vi "Launch Valves.vi"(8 "error in (no error)":errorcluster, 11 "Sample Line in":refnum<class "Sample Line.lvclass">) -> (0 "error out":errorcluster, 3 "Sample Line out":refnum<class "Sample Line.lvclass">)   [LabVIEW 2015, in "cRIO-Carbondioxide.lvlib" / "CO2-Actor.lvlib" / "Sample Line.lvclass"]
doc: "(<B>Filename</B>: Actor Framework.lvlib:Actor.lvclass:Pre Launch Init.vi)\n\nDefines behavior that occurs after the Launch Actor method is invoked but before the actor's Actor Core method begins running.\n\nThe Pre Launch Init method is guaranteed to finish before the Launch Actor method returns to its caller and before the actor itself receives any messages. Any references that the Pre Launch Init method obtains are guaranteed to have the same lifetime as the actor itself. Any errors that the Pre Launch Init method returns will abort the launch.\n\nBy default, this method does nothing. A descendant class may override it to define behavior."
uses:
  Sample Line.lvclass
  Valve/Action.ctl
  <vilib>/ActorFramework/Actor/Actor.lvclass
  Sample Line.lvclass/Sample Line.ctl
  CO2 Actor/CO2 Actor.lvclass
  Valve/Valve.lvclass
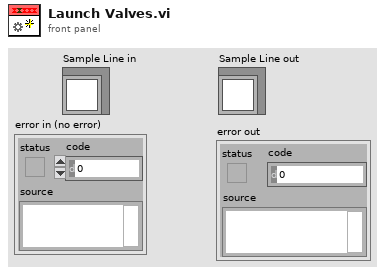
[diagram p1: front panel]
types:
  T1 = typedef "Action.ctl" = enum16{"Open", "Close", "None"}
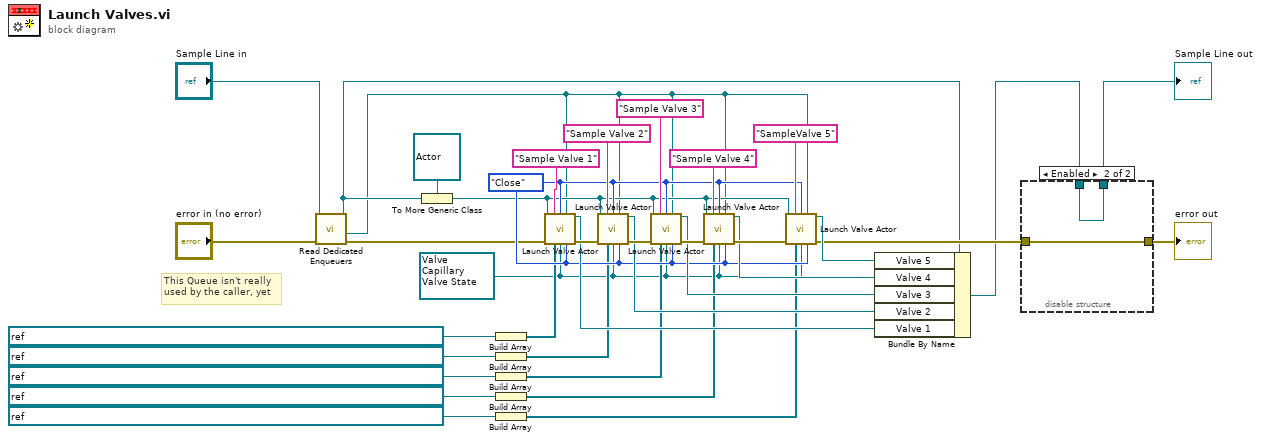
[diagram p0: block diagram]
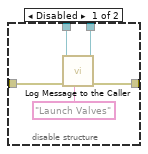
[diagram p2: hidden frame]
diagram:
  w3 = refnum<queue> refnum ("StateQ")
  w18 = Action."Close" ("Start Action (Open)")
  # "This Queue isn't really\nused by the caller, yet"
  n1 = call "Read Dedicated Enqueuers.vi"("error in (no error)"="error in (no error)", "CO2 Actor in"="Sample Line in") -> ("error out"=w5:errorcluster, "DedicatedEnQrs"=w1:refnum<queue>, "CO2 Actor out"=w2:refnum<class "Sample Line.lvclass">)  [unwired: 6 in, 1 out]
  n2 = To More Generic Class(target class=refnum<class "Actor.lvclass"> refnum ("Caller Actor in"), reference=w2) -> (generic class reference=w8:refnum<class "Actor.lvclass">)
  n3 = Build Array(refnum<k21> "ni.var.psp://10.2.0.20/AMS Gas SHV/Valves/Sample Line Valves/Sample Line 1" ("SHV")) -> (w13:refnum<k21>[])
  n4 = Build Array(refnum<k21> "ni.var.psp://10.2.0.20/AMS Gas SHV/Valves/Sample Line Valves/Sample Line 2" ("SHV")) -> (w12:refnum<k21>[])
  n5 = Build Array(refnum<k21> "ni.var.psp://10.2.0.20/AMS Gas SHV/Valves/Sample Line Valves/Sample Line 3" ("SHV")) -> (w11:refnum<k21>[])
  n6 = Build Array(refnum<k21> "ni.var.psp://10.2.0.20/AMS Gas SHV/Valves/Sample Line Valves/Sample Line 4" ("SHV")) -> (w10:refnum<k21>[])
  n7 = Build Array(refnum<k21> "ni.var.psp://10.2.0.20/AMS Gas SHV/Valves/Sample Line Valves/Sample Line 5" ("SHV")) -> (w9:refnum<k21>[])
  n8 = call "Launch Valve Actor.vi"("Caller Actor in"=w8, "Name"="Sample Valve 1", "Start Action (Open)"=w18, "DedicatedEnQrs"=w1, "error in (no error)"=w5, "SHV"=w13, "StateQ"=w3, "Stop Action (Close)"=w18) -> ("Caller-To-Actor Enqueuer"=w23:refnum<class "Message Enqueuer.lvclass">, "error out"=w36:errorcluster)  [unwired: 6 in]
  n9 = call "Launch Valve Actor.vi"("Caller Actor in"=w8, "Name"="Sample Valve 2", "Start Action (Open)"=w18, "DedicatedEnQrs"=w1, "error in (no error)"=w36, "SHV"=w12, "StateQ"=w3, "Stop Action (Close)"=w18) -> ("Caller-To-Actor Enqueuer"=w22:refnum<class "Message Enqueuer.lvclass">, "error out"=w35:errorcluster)  [unwired: 6 in]
  n10 = call "Launch Valve Actor.vi"("Caller Actor in"=w8, "Name"="Sample Valve 3", "Start Action (Open)"=w18, "DedicatedEnQrs"=w1, "error in (no error)"=w35, "SHV"=w11, "StateQ"=w3, "Stop Action (Close)"=w18) -> ("Caller-To-Actor Enqueuer"=w21:refnum<class "Message Enqueuer.lvclass">, "error out"=w34:errorcluster)  [unwired: 6 in]
  n11 = call "Launch Valve Actor.vi"("Caller Actor in"=w8, "Name"="Sample Valve 4", "Start Action (Open)"=w18, "DedicatedEnQrs"=w1, "error in (no error)"=w34, "SHV"=w10, "StateQ"=w3, "Stop Action (Close)"=w18) -> ("Caller-To-Actor Enqueuer"=w20:refnum<class "Message Enqueuer.lvclass">, "error out"=w37:errorcluster)  [unwired: 6 in]
  n12 = call "Launch Valve Actor.vi"("Caller Actor in"=w8, "Name"="SampleValve 5", "Start Action (Open)"=w18, "DedicatedEnQrs"=w1, "error in (no error)"=w37, "SHV"=w9, "StateQ"=w3, "Stop Action (Close)"=w18) -> ("Caller-To-Actor Enqueuer"=w19:refnum<class "Message Enqueuer.lvclass">, "error out"=w17:errorcluster)  [unwired: 6 in]
  n13 = Bundle By Name(cluster=w2, "Valve 5"=w19, "Valve 4"=w20, "Valve 3"=w21, "Valve 2"=w22, "Valve 1"=w23) -> (w15:refnum<class "Sample Line.lvclass">)
  n14 = disable-structure shown="Enabled" {
    disable-tunnel: w17 -> [w42 w44]
    disable-tunnel: [w41 w44] -> w16
    disable-tunnel: w15 -> [w40 w43]
    disable-tunnel: [w39 w43] -> w14
    frame Disabled {
      n15 = call-dynamic "Log Message to the Caller.vi"("String (\"\" = no message to send)"="Launch Valves" ("String (\"OK\")"), "error in (no error)"=w42, "CO2 Actor in"=w40) -> ("error out"=w41:errorcluster, "CO2 Actor out"=w39:refnum<class "Sample Line.lvclass">)  [unwired: 7 in]
    }
    frame Enabled {
    }
  }
  "error out" <- w16
  "Sample Line out" <- w14
